vi "UMLEditor SyncCodeFromUml.vi"(7 "Don't Prompt (False)":bool, 8 "error in":errorcluster, 10 "graph":refnum<class "Graph.lvclass">, 11 "selectedNode":refnum<class "AbstractNode.lvclass">) -> (0 "error out":errorcluster)   [LabVIEW 2020]
uses:
  <resource>/Framework/Providers/Open_GDS/UML/AbstractNode_class/AbstractNode.lvclass
  <resource>/Framework/Providers/Open_GDS/UML/Graph_class/Graph.lvclass
  <resource>/Framework/Providers/Open_GDS/UML/ClassNode_class/ExternalSetTypes.ctl
  <resource>/Framework/Providers/Open_GDS/UML/ClassNode_class/ClassNode.lvclass
  C:/Program Files (x86)/National Instruments/LabVIEW 2020/resource/Framework/Providers/Open_GDS/UML/AbstractNode_class/AbstractNode.lvclass
  <resource>/Framework/Providers/Open_GDS/ClassProviders/Common/CommonVIs/CommonVIs_ClassNamePathType.ctl
  <resource>/Framework/Providers/Open_GDS/UML/ClassRelationshipEdge_class/ClassRelationshipEdge.lvclass
  <resource>/Framework/Providers/Open_GDS/UML/AbstractEdge_class/AbstractEdge.lvclass
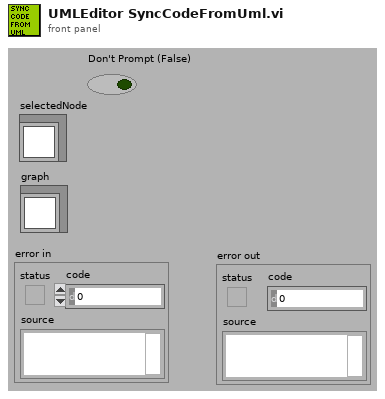
[diagram p1: front panel]
types:
  T1 = typedef "ClassNode.lvclass/ExternalSetTypes.ctl" = enum16{"Name", "Attributes", "Methods", "Position", "ShowMethods", "ShowAttributes", "ClassPath"}
  T2 = typedef "CommonVIs_ClassNamePathType.ctl" = cluster{"ClassNamn":string, "ClassPath":path, "InterfaceClass":bool}
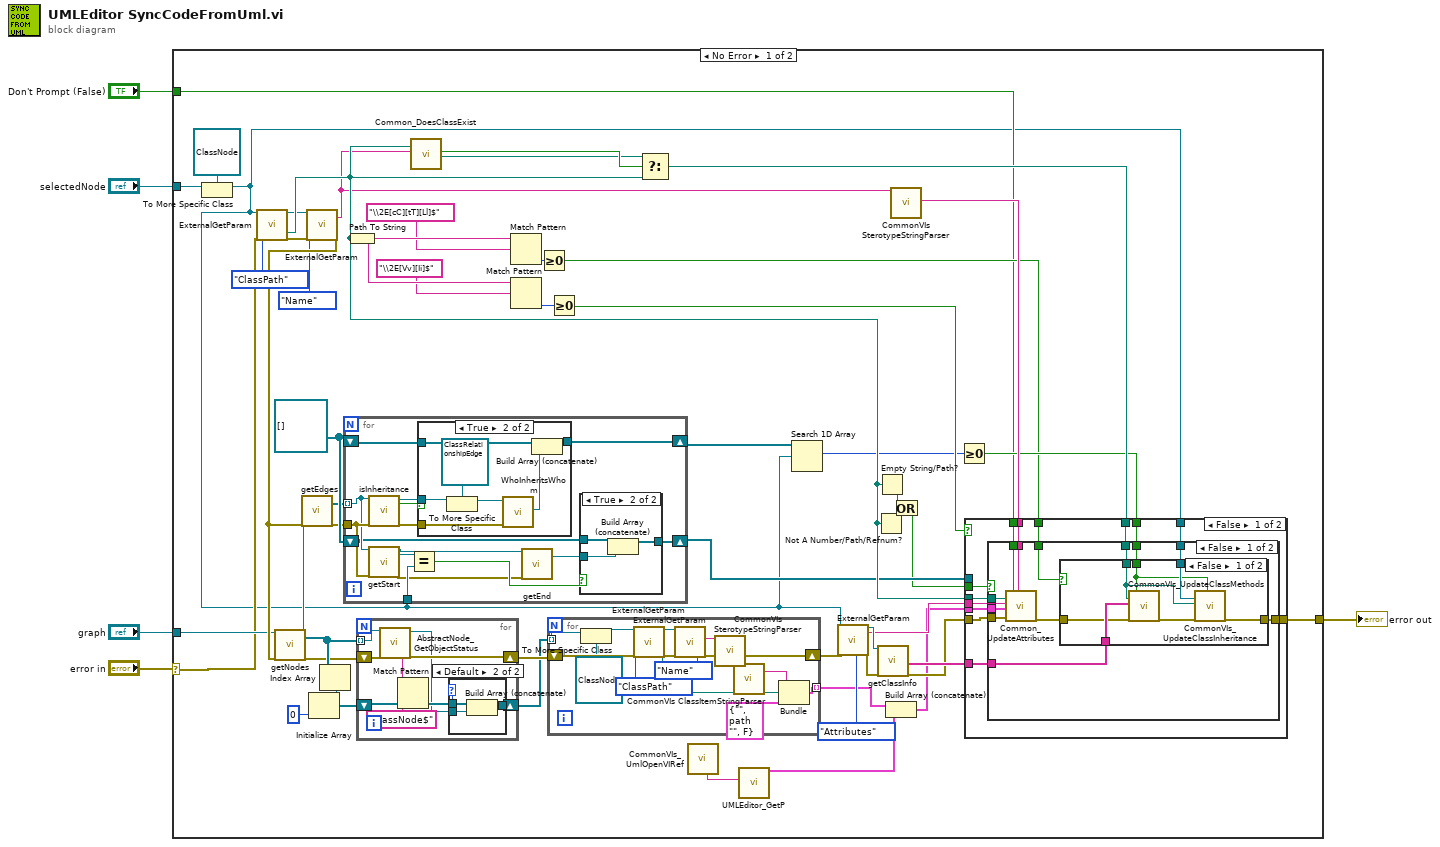
[diagram p0: block diagram]
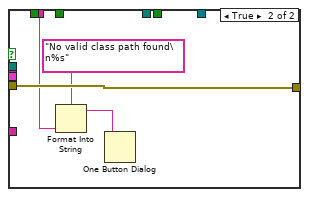
[diagram p3: hidden frame]
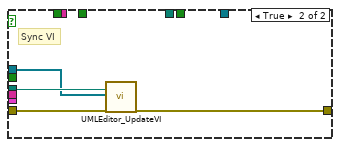
[diagram p4: hidden frame]
diagram:
  n1 = case shown="No Error" "error in" {
    selector: "error in" -> [w7 w157]
    tunnel: [w37 w157] -> w5
    tunnel: "graph" -> [w21 _]
    tunnel: "Don't Prompt (False)" -> [w14 _]
    tunnel: "selectedNode" -> [w8 _]
    frame No Error {
      w57 = refnum<class "AbstractNode.lvclass">[] []
      n2 = To More Specific Class(target class=refnum<class "ClassNode.lvclass"> refnum ("reference"), reference=w8) -> (specific class reference=w6:refnum<class "ClassNode.lvclass">)  [unwired: 1 in, 1 out]
      n3 = call <resource>:"ExternalGetParam.vi"("reference"=w6, "setParameter"=ExternalSetTypes."ClassPath", "error in (no error)"=w7) -> ("reference out"=w38:refnum<class "ClassNode.lvclass">, "Path"=w59:path, "error out"=w39:errorcluster)  [unwired: 14 out]
      n4 = call <resource>:"ExternalGetParam.vi"("reference"=w38, "setParameter"=ExternalSetTypes."Name", "error in (no error)"=w39) -> ("string"=w49:string, "error out"=w41:errorcluster)  [unwired: 15 out]
      n5 = call-dynamic "getNodes.vi"("reference"=w21, "error in (no error)"=w41) -> ("reference out"=w42:refnum<class "Graph.lvclass">, "nodes"=w20:refnum<class "AbstractNode.lvclass">[], "error out"=w19:errorcluster)  [unwired: 15 in]
      n6 = call-dynamic "getEdges.vi"("reference"=w42, "error in (no error)"=w41) -> ("edges"=w44:refnum<class "AbstractEdge.lvclass">[], "error out"=w43:errorcluster)  [unwired: 15 in, 1 out]
      n7 = Index Array(array=w20) -> (element=w16:refnum<class "AbstractNode.lvclass">)  [unwired: 1 in]
      n8 = Initialize Array(w16, 0 ("dimension size")) -> (w18:refnum<class "AbstractNode.lvclass">[])
      n9 = for {
        tunnel: w43 -> [w111]
        tunnel: w44 -> [w110] mode=indexing
        shift-right: [w113] -> w45
        shift-left: w57 -> [w114]
        tunnel: w6 -> [w109]
        shift-right: [w102] -> w58
        shift-left: w57 -> [w104]
        n10 = call-dynamic "isInheritance.vi"("reference"=w110, "error in (no error)"=w111) -> ("reference out"=w112:refnum<class "AbstractEdge.lvclass">, "isInheritance"=w115:bool, "error out"=w116:errorcluster)  [unwired: 13 in, 2 out]
        n11 = call-dynamic "getStart.vi"("reference"=w110, "error in (no error)"=w111) -> ("reference out"=w105:refnum<class "AbstractEdge.lvclass">, "startNode"=w108:refnum<class "AbstractNode.lvclass">, "error out"=w106:errorcluster)  [unwired: 14 in, 1 out]
        n12 = Equal?(x=w108, y=w109) -> (x = y?=w107:bool)
        n13 = case shown="True" w115 {
          tunnel: w116 -> [_ w128]
          tunnel: w114 -> [w121 w127]
          tunnel: [w121 w125] -> w113
          tunnel: w112 -> [_ w124]
          frame False {
          }
          frame True {
            n14 = To More Specific Class(target class=refnum<class "ClassRelationshipEdge.lvclass"> refnum ("reference"), reference=w124) -> (specific class reference=w122:refnum<class "ClassRelationshipEdge.lvclass">)  [unwired: 1 in, 1 out]
            n15 = call <resource>:"WhoInheritsWhom.vi"("reference"=w122, "error in (no error)"=w128) -> ("base"=w126:refnum<class "AbstractNode.lvclass">)  [unwired: 17 out]
            n16 = Build Array (concatenate)(w127, w126) -> (w125:refnum<class "AbstractNode.lvclass">[])
          }
        }
        n17 = call-dynamic "getEnd.vi"("reference"=w105, "error in (no error)"=w106) -> ("endNode"=w103:refnum<class "AbstractNode.lvclass">)  [unwired: 14 in, 3 out]
        n18 = case shown="True" w107 {
          tunnel: w104 -> [w117 w120]
          tunnel: w103 -> [_ w119]
          tunnel: [w117 w118] -> w102
          frame False {
          }
          frame True {
            n19 = Build Array (concatenate)(w120, w119) -> (w118:refnum<class "AbstractNode.lvclass">[])
          }
        }
      }
      n20 = Path To String(path=w59) -> (string=w55:string)
      n21 = for {
        shift-right: [w150] -> w23
        shift-left: w19 -> [w152]
        tunnel: w20 -> [w151] mode=indexing
        shift-right: [w147] -> w22
        shift-left: w18 -> [w149]
        n22 = call <resource>:"AbstractNode_GetObjectStatus.vi"("reference in"=w151, "error in (no error)"=w152) -> ("Class name"=w146:string, "reference out"=w148:refnum<class "AbstractNode.lvclass">, "error out"=w150:errorcluster)  [unwired: 15 out]
        n23 = Match Pattern(string=w146, regular expression="ClassNode$") -> (offset past match=w144:i32)  [unwired: 4 out]
        n24 = case shown="Default" w144 {
          tunnel: w149 -> [w153 w156]
          tunnel: w148 -> [_ w155]
          tunnel: [w153 w154] -> w147
          frame -1 {
          }
          frame Default {
            n25 = Build Array (concatenate)(w156, w155) -> (w154:refnum<class "AbstractNode.lvclass">[])
          }
        }
      }
      n26 = call <resource>:"Common_DoesClassExist.vi"("ClassPath"=w59, "ClassName"=w49) -> ("llb-class"=w51:bool, "llb/LvCLass-Path"=w50:path)  [unwired: 16 out]
      n27 = Match Pattern(string=w55, regular expression="\\2E[cC][tT][Ll]$") -> (offset past match=w27:i32)  [unwired: 4 out]
      n28 = Match Pattern(string=w55, regular expression="\\2E[Vv][Ii]$") -> (offset past match=w53:i32)  [unwired: 4 out]
      n29 = Greater Or Equal To 0?(x=w27) -> (x >= 0?=w33:bool)
      n30 = for {
        tunnel: w22 -> [w131] mode=indexing
        shift-right: [w138] -> w24
        shift-left: w23 -> [w142]
        tunnel: [w137] -> w10 mode=indexing
        n31 = To More Specific Class(target class=refnum<class "ClassNode.lvclass"> refnum ("reference"), reference=w131) -> (specific class reference=w130:refnum<class "ClassNode.lvclass">)  [unwired: 1 in, 1 out]
        n32 = call <resource>:"ExternalGetParam.vi"("reference"=w130, "setParameter"=ExternalSetTypes."ClassPath", "error in (no error)"=w142) -> ("reference out"=w139:refnum<class "ClassNode.lvclass">, "Path"=w135:path, "error out"=w141:errorcluster)  [unwired: 14 out]
        n33 = call <resource>:"ExternalGetParam.vi"("reference"=w139, "setParameter"=ExternalSetTypes."Name", "error in (no error)"=w141) -> ("string"=w136:string, "error out"=w138:errorcluster)  [unwired: 15 out]
        n34 = call <resource>:"CommonVIs SterotypeStringParser.vi"("SterotypeStringIn"=w136) -> ("Name"=w134:string)  [unwired: 18 out]
        n35 = call <resource>:"CommonVIs ClassItemStringParser.vi"("ClassItemNameIn"=w134) -> ("Name"=w133:string)  [unwired: 18 out]
        n36 = Bundle(cluster=T2 {"ClassNamn"="", "ClassPath"=path "", "InterfaceClass"=FALSE} ("Cluster"), "ClassNamn"=w133, "ClassPath"=w135) -> (w137:T2)  [unwired: 1 in]
      }
      n37 = Greater Or Equal To 0?(x=w53) -> (x >= 0?=w56:bool)
      n38 = Select(t=w50, s=w51, f=w59) -> (s? t:f=w52:path)
      n39 = call <resource>:"CommonVIs_UmlOpenVIRef.vi"() -> ("ProjectNameOut"=w13:string)  [unwired: 4 in, 7 out]
      n40 = call <resource>:"UMLEditor_GetP.vi"("GetProjectRefByName/or Ref"=w13) -> ("ClassesNamesAndPaths"=w12:T2[])  [unwired: 1 in, 9 out]
      n41 = Search 1D Array(1D array=w45, element=w6) -> (index of element=w46:i32)  [unwired: 1 out]
      n42 = call <resource>:"ExternalGetParam.vi"("reference"=w6, "setParameter"=ExternalSetTypes."Attributes", "error in (no error)"=w24) -> ("reference out"=w35:refnum<class "ClassNode.lvclass">, "string"=w34:string, "error out"=w36:errorcluster)  [unwired: 14 out]
      n43 = Not A Number/Path/Refnum?(number/path/refnum=w59) -> (NaN/Path/Refnum?=w29:bool)
      n44 = Empty String/Path?(string/path=w59) -> (empty?=w28:bool)
      n45 = call-dynamic "getClassInfo.vi"("reference"=w35, "error in (no error)"=w36) -> ("methods"=w32:string[], "error out"=w31:errorcluster)  [unwired: 8 in, 8 out]
      n46 = Build Array (concatenate)(w10, w12) -> (w11:T2[])
      n47 = call <resource>:"CommonVIs SterotypeStringParser.vi"("SterotypeStringIn"=w49) -> ("Sterotype"=w48:string)  [unwired: 18 out]
      n48 = Or(x=w28, y=w29) -> (x .or. y?=w30:bool)
      n49 = Greater Or Equal To 0?(x=w46) -> (x >= 0?=w47:bool)
      n50 = case shown="False" w56 {
        tunnel: w30 -> [w72 _]
        tunnel: w31 -> [w71 w101]
        tunnel: w32 -> [w70 _]
        tunnel: w59 -> [w69 w99]
        tunnel: w33 -> [w68 _]
        tunnel: w11 -> [w67 _]
        tunnel: w34 -> [w66 _]
        tunnel: [w65 w100] -> w37
        tunnel: w47 -> [w64 _]
        tunnel: w48 -> [w63 _]
        tunnel: w52 -> [w62 _]
        tunnel: w58 -> [_ w98]
        tunnel: w14 -> [w61 _]
        tunnel: w6 -> [w60 _]
        frame False {
          n51 = case shown="False" w72 {
            tunnel: [w80 w97] -> w65
            tunnel: w66 -> [w85 _]
            tunnel: w71 -> [w84 w97]
            tunnel: w67 -> [w83 _]
            tunnel: w69 -> [w82 _]
            tunnel: w68 -> [w79 _]
            tunnel: w62 -> [w78 _]
            tunnel: w70 -> [w77 _]
            tunnel: w64 -> [w76 _]
            tunnel: w63 -> [w75 w94]
            tunnel: w61 -> [w74 _]
            tunnel: w60 -> [w73 _]
            frame False {
              n52 = call <resource>:"Common_UpdateAttributes.vi"("ClassPath/LvClassRef"=w82, "NewAttributes"=w85, "ClassInfo"=w83, "error in (no error)"=w84, "Don't Prompt (False)"=w74, "Stereotype"=w75) -> ("error out"=w81:errorcluster)  [unwired: 13 out]
              n53 = case shown="False" w79 {
                tunnel: w81 -> [w90 w93]
                tunnel: [w89 w93] -> w80
                tunnel: w78 -> [w87 _]
                tunnel: w77 -> [w91 _]
                tunnel: w76 -> [w86 _]
                tunnel: w73 -> [w88 _]
                frame False {
                  n54 = call <resource>:"CommonVIs_UpdateClassMethods.vi"("ClassPath/LvClassRef"=w87, "Methods"=w91, "error in (no error)"=w90, "BaseClass"=w86) -> ("error out"=w92:errorcluster)  [unwired: 3 in, 12 out]
                  n55 = call <resource>:"CommonVIs_UpdateClassInheritance.vi"("ClassNodeToAnalyse"=w88, "ClassPath/LvClassRef"=w87, "error in (no error)"=w92, "UseVirtualMethods(True)"=w86) -> ("error out"=w89:errorcluster)  [unwired: 15 in]
                }
                frame True {
                }
              }
            }
            frame True {
              n56 = Format Into String(format string="No valid class path found\n%s" ("message"), w94) -> (resulting string=w95:string)  [unwired: 2 in, 1 out]
              n57 = One Button Dialog(message=w95) -> ()  [unwired: 2 out]
            }
          }
        }
        frame True {
          # "Sync VI"
          n58 = call <resource>:"UMLEditor_UpdateVI.vi"("ViPath"=w99, "DependendClasses"=w98, "error in (no error)"=w101) -> ("error out"=w100:errorcluster)  [unwired: 16 out]
        }
      }
    }
    frame Error {
    }
  }
  "error out" <- w5
